vi "Z900_navX_Util_EncodeProtocol_Int16.vi"(1 "Int16":i16[](array[numeric])) -> (0 "Little Endian":u8[](array[numeric]))   [LabVIEW 2019, in "navX Library v2.lvlib"]
uses:
  navX Library v2.lvlib
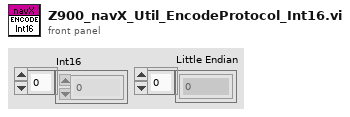
[diagram p1: front panel]
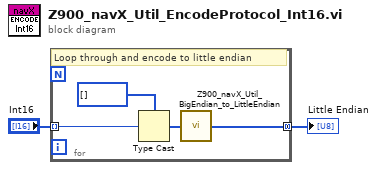
[diagram p0: block diagram]
diagram:
  n1 = for {
    tunnel: "Int16" -> [w6] mode=indexing
    tunnel: [w3] -> w1 mode=concatenating
    # "Loop through and encode to little endian"
    n2 = Type Cast(type=u8[] [], x=w6) -> (*(type *) &x=w4:u8[])
    n3 = call "Z900_navX_Util_BigEndian_to_LittleEndian.vi"("Big Endian"=w4) -> ("Little Endian"=w3:u8[])
  }
  "Little Endian" <- w1
